vi "StartClone.vi"(7 "ShowPanel? (F)":bool, 8 "error in (no error)":errorcluster, 10 "ModuleName":string="unnamed", 11 "VI Refnum":refnum<vi>) -> (0 "error out":errorcluster, 1 "FGenBroadcast":T1, 3 "ModuleAdmin":refnum<class "ModuleAdmin.lvclass">)   [LabVIEW 2014, in "FGenModule.lvlib"]
uses:
  FGenModule.lvlib
  Protected/Broadcasts/clBroadcastEvents.ctl
  Protected/clEventType.ctl
  <userlib>/NIST/ModuleAdminLib/ModuleAdmin/ModuleAdmin.lvclass
  <userlib>/NIST/ModuleAdminLib/ModuleAdmin/ModuleAdmin.lvclass/ModuleAdmin.ctl
  <userlib>/NIST/ModuleAdminLib/ModuleAdmin/Accessors/Write CloneRegRef.vi
  <userlib>/NIST/ModuleAdminLib/ModuleAdmin/Accessors/Write ShowPanel_.vi
  <vilib>/Utility/error.llb/Error Cluster From Error Code.vi
  <vilib>/ErrorRing/Error Ring.xnode
  <userlib>/NIST/ModuleAdminLib/CloneRegistration/CloneRegistration.lvclass
panel:
  # "If you want to add other Broadcast Events, open this typedef, copy an existing event and rename it to your event name.\n\nNext create an \"arg\" typedef for the  data and put it into PublicAPI/Arguments/Broadcasts\n\nAfter that, you will need to create a new roadcast vi in Protected/Broadcast.  Look at DidInit.vi or the reportError.vi as examples."
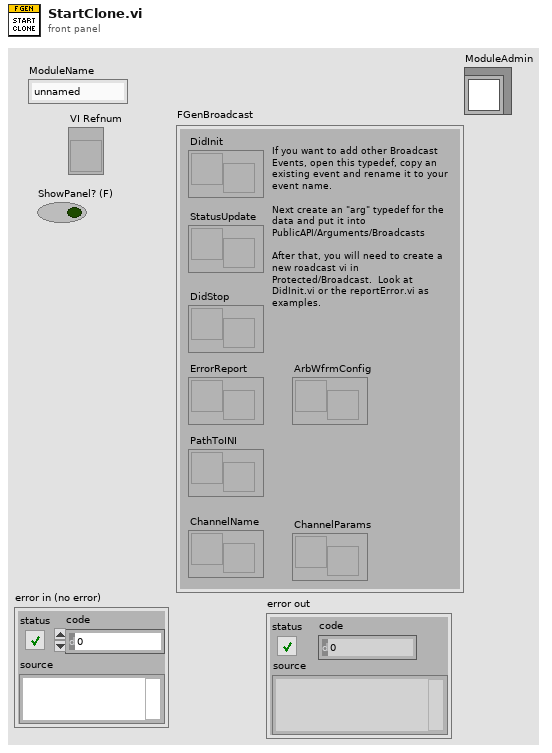
[diagram p1: front panel]
types:
  T1 = typedef "FGenModule.lvlib/clBroadcastEvents.ctl" = cluster{"DidInit":refnum<user-event>, "StatusUpdate":refnum<user-event>, "ErrorReport":refnum<user-event>, "DidStop":refnum<user-event>, "PathToINI":refnum<user-event>, "ChannelName":refnum<user-event>, "ArbWfrmConfig":refnum<user-event>, "ChannelParams":refnum<user-event>}
  T2 = enum32{"Bad", "Idle", "Run top level", "Running"}
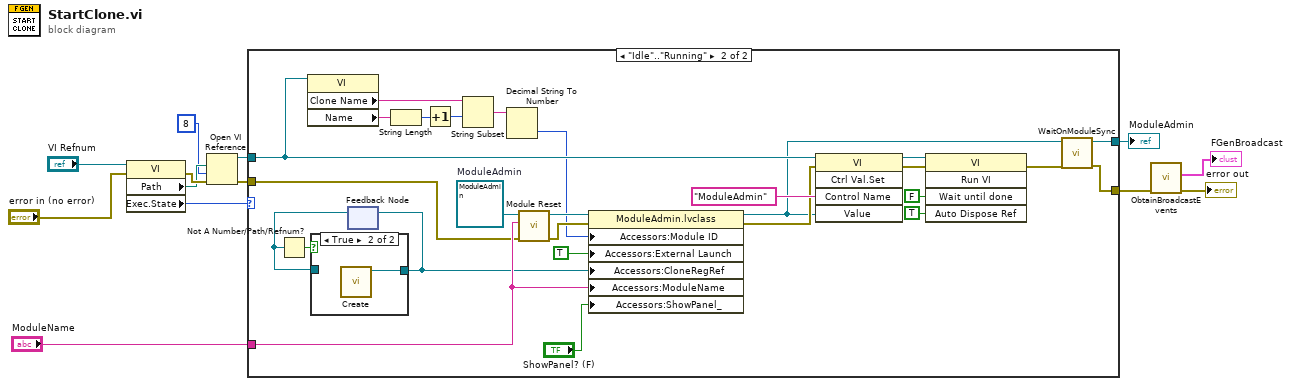
[diagram p0: block diagram]
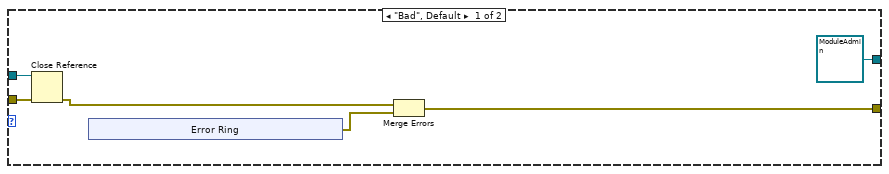
[diagram p2: hidden frame]
diagram:
  n1 = property class="VI"(reference="VI Refnum", error in="error in (no error)") -> (error out=w11:errorcluster, "Path"=w10:path, "Exec.State"=w12:T2)  [unwired: 1 out]
  n2 = Open VI Reference(vi path=w10, options=8, error in (no error)=w11) -> (vi reference=w8:refnum<vi>, error out=w9:errorcluster)  [unwired: 3 in]
  n3 = case shown="\"Idle\"..\"Running\"" w12 {
    tunnel: w9 -> [w19 w24]
    tunnel: w8 -> [w18 w41]
    tunnel: [w15 w31] -> w5
    tunnel: "ModuleName" -> [_ w30]
    tunnel: [refnum<class "ModuleAdmin.lvclass"> refnum ("ModuleAdmin") w29] -> w1
    frame "Bad", Default {
      n4 = Close Reference(reference=w18, error in (no error)=w19) -> (error out=w17:errorcluster)
      n5 = xnode "Error Ring"() -> ("error out"=w16:errorcluster)
      n6 = Merge Errors(w17, w16) -> (w15:errorcluster)
    }
    frame "Idle".."Running" {
      w45 = refnum<class "ModuleAdmin.lvclass"> refnum  # ModuleAdmin
      n7 = property class="VI"(reference=w41) -> ("Clone Name"=w47:string, "Name"=w50:string)  [unwired: 1 in, 2 out]
      n8 = feedback #1() -> (w26:refnum<data-value>)  [unwired: 1 in]
      n9 = Not A Number/Path/Refnum?(number/path/refnum=w26) -> (NaN/Path/Refnum?=w27:bool)
      n10 = case shown="True" w27 {
        tunnel: [w51 w52] -> w25
        tunnel: w26 -> [w51 _]
        frame False {
        }
        frame True {
          n11 = call <userlib>:"Create.vi"() -> ("CloneRegRef"=w52:refnum<data-value>)  [unwired: 10 in, 1 out]
        }
      }
      n12 = feedback-in #1(w25) -> ()
      n13 = String Length(string=w50) -> (length=w49:i32)
      n14 = Increment(x=w49) -> (x+1=w48:i32)
      n15 = String Subset(string=w47, offset (0)=w48) -> (substring=w46:string)  [unwired: 1 in]
      n16 = Decimal String To Number(string=w46) -> (number=w33:i32)  [unwired: 2 in, 1 out]
      n17 = call <userlib>:"Module Reset.vi"("error in (no error)"=w24, "ModuleName"=w30, "Mod Admin in"=w45) -> ("error out"=w44:errorcluster, "Mod Admin out"=w43:refnum<class "ModuleAdmin.lvclass">)  [unwired: 7 in]
      n18 = property class="ModuleAdmin.lvclass"(reference=w43, error in=w44, "Accessors:Module ID"=w33, "Accessors:External Launch"=TRUE ("External Launch"), "Accessors:CloneRegRef"=w25, "Accessors:ModuleName"=w30, "Accessors:ShowPanel_"="ShowPanel? (F)") -> (reference out=w32:refnum<class "ModuleAdmin.lvclass">, error out=w34:errorcluster)
      n19 = invoke class="VI" method="Ctrl Val.Set"(reference=w41, error in=w34, "Control Name"="ModuleAdmin", "Value"=w32) -> (reference out=w39:refnum<vi>, error out=w38:errorcluster)  [unwired: 1 in, 3 out]
      n20 = invoke class="VI" method="Run VI"(reference=w39, error in=w38, "Wait until done"=FALSE ("Wait Until Done"), "Auto Dispose Ref"=TRUE ("Auto Dispose Reference")) -> (error out=w35:errorcluster)  [unwired: 1 in, 4 out]
      n21 = call <userlib>:"WaitOnModuleSync.vi"("error in (no error)"=w35, "ModuleAdmin"=w32) -> ("error out"=w31:errorcluster, "ModuleAdmin"=w29:refnum<class "ModuleAdmin.lvclass">)  [unwired: 8 in]
    }
  }
  "ModuleAdmin" <- w1
  n22 = call "ObtainBroadcastEvents.vi"("error in (no error)"=w5) -> ("error out"=→"error out":errorcluster, "clBroadcastEvents"=→"FGenBroadcast":T1)  [unwired: 9 in]
